vi "Jog.vi"(4 "One Axis Rel Distanz mm":dbl, 6 "Rel. Move Type":bool=TRUE, 8 "error in (no error)":errorcluster, 9 "Axis (1..4)":T1=1 items=["X"=1, "Y"=2, "Z"=3, "T"=4], 10 "Direction -1, 1":i32, 11 "VXMx2 in":refnum<class "VXMx2.lvclass">) -> (0 "error out":errorcluster, 3 "VXMx2 out":refnum<class "VXMx2.lvclass">, 5 "Position, eng units":dbl)   [LabVIEW 2019, in "VXMx2.lvclass"]
doc: "send relative move command, wait until motion stops."
uses:
  VXMx2.lvclass
  <instrlib>/Velmex VXM/Public/VXM Axis.ctl
  Support/MessageAPI/UIMessage.ctl
  VXMx2.lvclass/VXMx2.ctl
  SendMessage/SendMessage.lvclass
  <instrlib>/Velmex VXM/Velmex VXM.lvlib
panel:
  out "i":i32
  out "Limit Switch Activated":bool
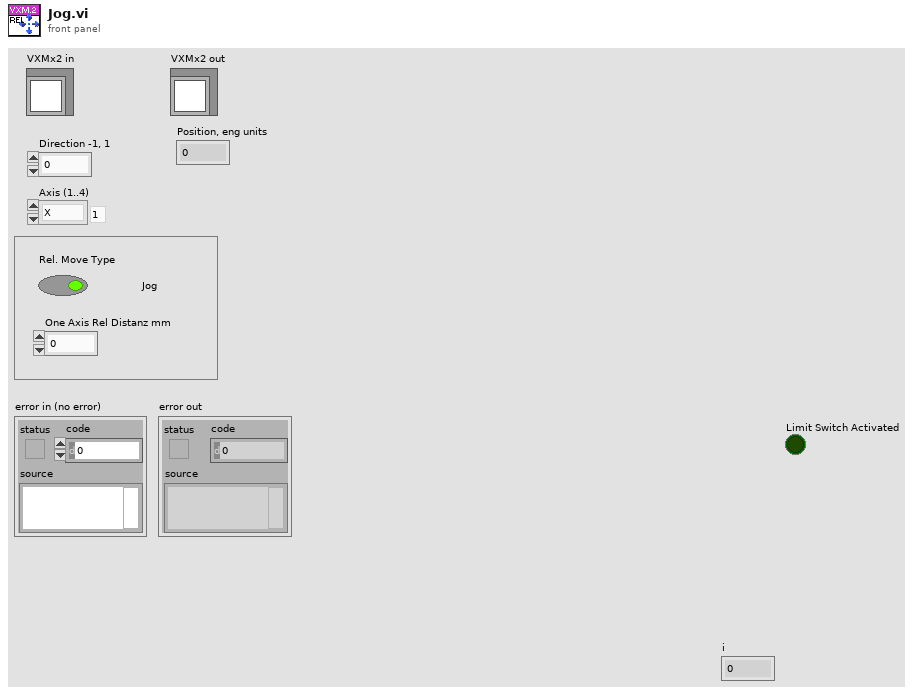
[diagram p1: front panel]
types:
  T1 = typedef "Velmex VXM.lvlib/VXM Axis.ctl" = u16
  T2 = typedef "UIMessage.ctl" = cluster{"EventCode":i32, "Numeric":dbl, "String":string, "Variant":variant}
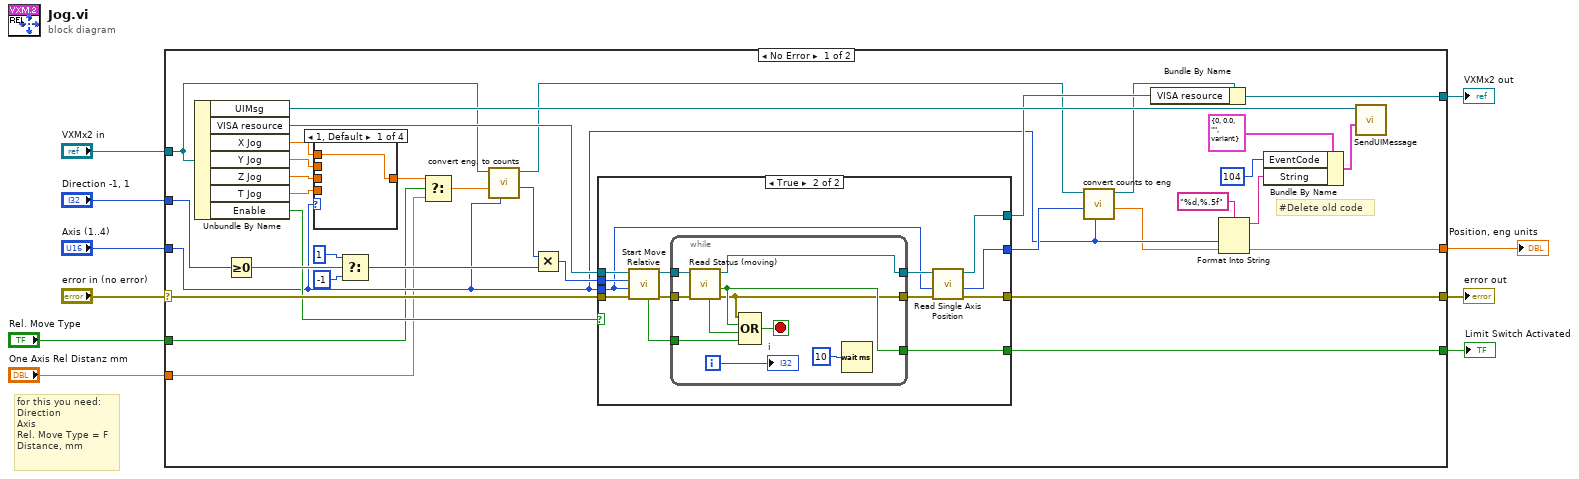
[diagram p0: block diagram]
diagram:
  # "for this you need:\nDirection\nAxis\nRel. Move Type = F\nDistance, mm"
  n1 = case shown="No Error" "error in (no error)" {
    selector: "error in (no error)" -> [w33 w76]
    tunnel: [w24 w76] -> w9
    tunnel: [w26 w75] -> w7
    tunnel: "VXMx2 in" -> [w18 w75]
    tunnel: "Axis (1..4)" -> [w16 _]
    tunnel: "Direction -1, 1" -> [w38 _]
    tunnel: [w23 _] -> w4
    tunnel: "Rel. Move Type" -> [w13 _]
    tunnel: "One Axis Rel Distanz mm" -> [w12 _]
    tunnel: [w11 _] -> w1
    frame No Error {
      # "#Delete old code"
      n2 = Unbundle By Name(w18) -> ("UIMsg"=w27:refnum<class "SendMessage.lvclass">, "VISA resource"=w44:refnum<visa-resource-name>, "X Jog"=w43:dbl, "Y Jog"=w42:dbl, "Z Jog"=w41:dbl, "T Jog"=w40:dbl, "Enable"=w22:bool)
      n3 = Greater Or Equal To 0?(x=w38) -> (x >= 0?=w37:bool)
      n4 = case shown="1, Default" w16 {
        tunnel: [w71 w72 w73 w74] -> w14
        tunnel: w43 -> [w71 _ _ _]
        tunnel: w42 -> [_ w72 _ _]
        tunnel: w41 -> [_ _ w73 _]
        tunnel: w40 -> [_ _ _ w74]
        frame 1, Default {
        }
        frame 2 {
        }
        frame 3 {
        }
        frame 4 {
        }
      }
      n5 = Select(t=1 ("Direction"), s=w37, f=-1 ("Direction")) -> (s? t:f=w34:i32)
      n6 = Select(t=w14, s=w13, f=w12) -> (s? t:f=w15:dbl)
      n7 = call "convert eng. to counts.vi"("Axis (1..4)"=w16, "Position, eng units"=w15, "VXMx2 in"=w18) -> ("Position, counts"=w19:i32, "VXMx2 out"=w17:refnum<class "VXMx2.lvclass">)  [unwired: 5 in, 2 out]
      n8 = Multiply(x=w19, y=w34) -> (x*y=w39:i32)
      n9 = case shown="True" w22 {
        tunnel: w44 -> [w47 w60]
        tunnel: w39 -> [w46 w59]
        tunnel: w33 -> [w45 w56]
        tunnel: w16 -> [_ w53]
        tunnel: [w46 w52] -> w20
        tunnel: [w47 w49] -> w25
        tunnel: [w45 w51] -> w24
        tunnel: [_ w50] -> w23
        frame False {
        }
        frame True {
          n10 = call <instrlib>:"Start Move Relative.vi"("error in (no error)"=w56, "Axis (1..4)"=w53, "Relative Move, counts"=w59, "VISA resource name"=w60) -> ("error out"=w58:errorcluster, "VISA resource out"=w57:refnum<visa-resource-name>, "Relative Move = 0"=w48:bool)  [unwired: 5 in]
          n11 = while {
            tunnel: w58 -> [w67]
            tunnel: [w62] -> w55
            tunnel: w57 -> [w65]
            tunnel: [w64] -> w54
            tunnel: [w63] -> w50
            tunnel: w48 -> [w61]
            i -> [w69]
            stop <- w70 stop-if-true
            n12 = call <instrlib>:"Read Status (moving).vi"("error in (no error)"=w67, "VISA resource name"=w65) -> ("error out"=w62:errorcluster, "Limit Switch Activated"=w63:bool, "VISA resource out"=w64:refnum<visa-resource-name>, "Motion Stopped"=w66:bool)  [unwired: 5 in, 1 out]
            n13 = Compound Arithmetic op=OR(w62, w63, w66, w61) -> (w70:bool)
            n14 = Wait (ms)(milliseconds to wait=u32 10) -> ()  [unwired: 1 out]
            "i" <- w69
          }
          n15 = call <instrlib>:"Read Single Axis Position.vi"("error in (no error)"=w55, "Axis (1..4)"=w53, "VISA resource name"=w54) -> ("error out"=w51:errorcluster, "Position, counts"=w52:i32, "VISA resource out"=w49:refnum<visa-resource-name>)  [unwired: 6 in]
        }
      }
      n16 = call "convert counts to eng.vi"("Axis (1..4)"=w16, "Position, counts"=w20, "VXMx2 in"=w17) -> ("Position, eng units"=w11:dbl, "VXMx2 out"=w21:refnum<class "VXMx2.lvclass">)  [unwired: 5 in, 2 out]
      n17 = Bundle By Name(cluster=w21, "VISA resource"=w25) -> (w26:refnum<class "VXMx2.lvclass">)
      n18 = Format Into String(format string="%d,%.5f", w16, w11) -> (resulting string=w30:string)  [unwired: 2 in, 1 out]
      n19 = Bundle By Name(cluster=T2 {"EventCode"=0, "Numeric"=0.0, "String"="", "Variant"=variant} ("UIMsg"), "EventCode"=104, "String"=w30) -> (w29:T2)
      n20 = call-dynamic "SendUIMessage.vi"("UIMsg"=w29, "SendMessage in"=w27) -> ()  [unwired: 8 in, 2 out]
    }
    frame Error {
    }
  }
  "error out" <- w9
  "VXMx2 out" <- w7
  "Limit Switch Activated" <- w4
  "Position, eng units" <- w1
